vi "Lr3v3v15.vi"() -> ()   [LabVIEW 2012]
uses:
  <vilib>/express/express analysis/Spectral/Block/exnSpectralBlock spectral measurements power poly.vi
  <vilib>/express/express analysis/Spectral/Block/exnSpectralBlock spectral measurements power DDT.vi
  <vilib>/express/express analysis/Spectral/XNode/ExpressSpectralMeasurementsBlockNode.xnode
panel:
  out "Max":dbl
  out "Min":dbl
  out "RMS":dbl
  out "Colleration":dynamicdata(graph)
  out "Spectral":dynamicdata(graph)
  out "Histogram":dynamicdata(graph)
  in  "stop":bool
  in  "Filter":bool
  in  "A0":dbl(slide) scale=0.0..3.0
  in  "A":dbl(slide) scale=1.0..10.0
  in  "Hz":dbl(knob) scale=10.0..100.0
  in  "Time rag.":dbl(slide) scale=500.0..2000.0
  out "Waveform Graph":dynamicdata(graph)
  # "Highpass"
  # "Bandstop"
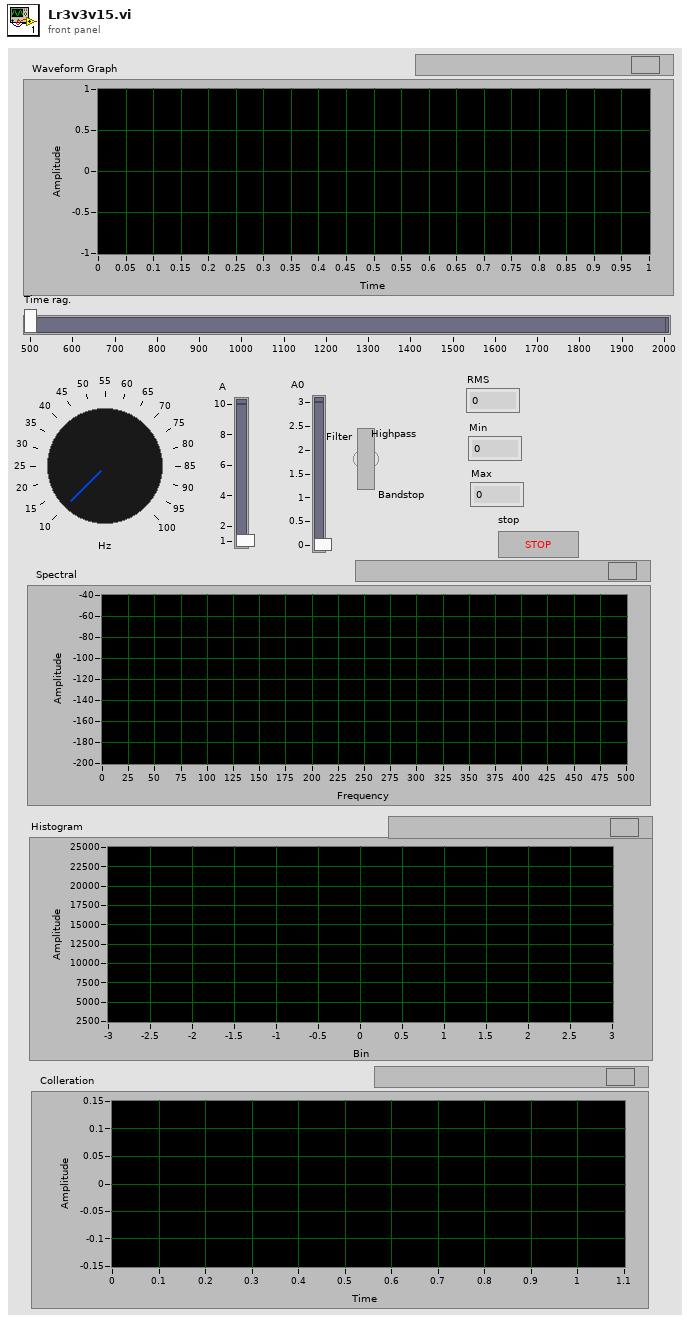
[diagram p1: front panel]
types:
  T1 = cluster{"averaging mode":u16, "weighting mode":u16, "number of averages":u32}
  T2 = cluster{"dB On (F)":bool, "unwrap phase (F)":bool, "convert to degree (F)":bool}
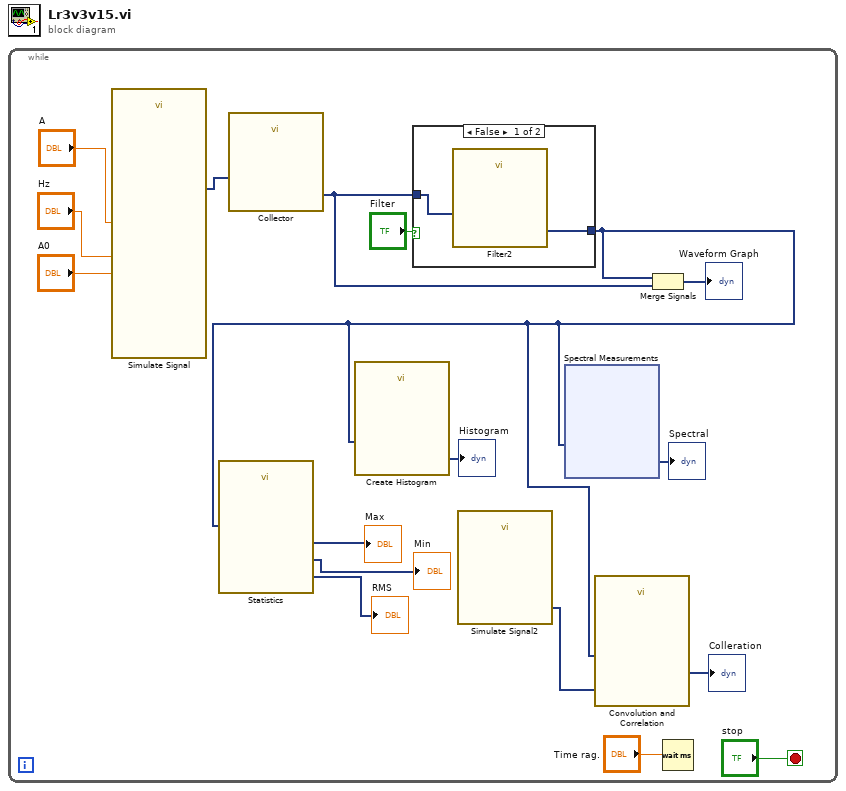
[diagram p0: block diagram]
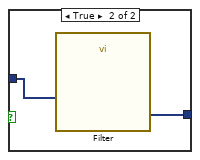
[diagram p2: hidden frame]
diagram:
  n1 = while {
    stop <- "stop" stop-if-true
    n2 = call "Simulate Signal"("Frequency"="Hz", "Amplitude"="A", "Noise amplitude"="A0") -> ("Sine with Uniform Noise"=w14:dynamicdata)  [unwired: 11 in, 1 out]
    n3 = call "Collector"("Signals"=w14) -> ("Collected Signals"=w11:dynamicdata)  [unwired: 9 in, 1 out]
    n4 = case shown="False" "Filter" {
      tunnel: w11 -> [w28 w30]
      tunnel: [w27 w29] -> w6
      frame False {
        n5 = call "Filter2"("Signal"=w28) -> ("Filtered Signal"=w27:dynamicdata)  [unwired: 9 in, 1 out]
      }
      frame True {
        n6 = call "Filter"("Signal"=w30) -> ("Filtered Signal"=w29:dynamicdata)  [unwired: 9 in, 1 out]
      }
    }
    n7 = call "Statistics"("Signals"=w6) -> ("RMS"=→"RMS":dynamicdata, "Minimum"=→"Min":dynamicdata, "Maximum"=→"Max":dynamicdata)  [unwired: 23 in, 1 out]
    n8 = call "Create Histogram"("Signal"=w6) -> ("Histogram"=→"Histogram":dynamicdata)  [unwired: 9 in, 1 out]
    n9 = call "Simulate Signal2"() -> ("Sine"=w5:dynamicdata)  [unwired: 14 in, 1 out]
    n10 = xnode "Spectral Measurements"("Signals"=w6) -> ("Power Spectrum"=→"Spectral":dynamicdata)  [unwired: 1 in, 1 out]
    n11 = call "Convolution and Correlation"("Y"=w5, "X"=w6) -> ("X*Y"=→"Colleration":dynamicdata)  [unwired: 8 in, 1 out]
    n12 = Merge Signals(w6, w11) -> (→"Waveform Graph":dynamicdata)
    n13 = Wait (ms)(milliseconds to wait="Time rag.") -> ()  [unwired: 1 out]
  }
